vi "input cyl-list output array.vi"(11 "cyl list":string[](array[string])) -> (3 "Array":u8[][](array[numeric]))   [LabVIEW 2011]
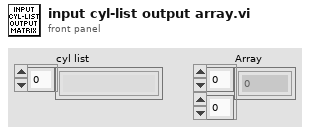
[diagram p1: front panel]
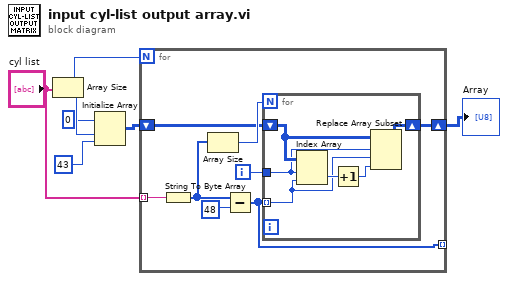
[diagram p0: block diagram]
diagram:
  n1 = Array Size(array="cyl list") -> (size(s)=w3:i32)
  n2 = Initialize Array(u8 0, w3, 43 ("dimension size")) -> (w5:u8[][])
  n3 = for {
    N: w3 -> [_]
    tunnel: "cyl list" -> [w14] mode=indexing
    shift-right: [w8] -> w6
    shift-left: w5 -> [w9]
    tunnel: [w7] -> _ mode=indexing
    i -> [w10]
    n4 = String To Byte Array(string=w14) -> (unsigned byte array=w12:u8[])
    n5 = Array Size(array=w12) -> (size(s)=w11:i32)
    n6 = Subtract(x=w12, y=u8 48) -> (x-y=w7:u8[])
    n7 = for {
      N: w11 -> [_]
      tunnel: w7 -> [w17] mode=indexing
      tunnel: w10 -> [w18]
      shift-right: [w15] -> w8
      shift-left: w9 -> [w19]
      n8 = Index Array(array=w19, index (row)=w18, index (col)=w17) -> (element=w20:u8)
      n9 = Increment(x=w20) -> (x+1=w16:u8)
      n10 = Replace Array Subset(array=w19, new element=w16, index (row)=w18, index (col)=w17) -> (w15:u8[][])
    }
  }
  "Array" <- w6
